vi "Store ASCII string.vi"(8 "error in (no error)":errorcluster, 10 "String to store (max 16 chars)":string, 11 "VISA resource name":refnum<visa-resource-name>) -> (0 "error out":errorcluster, 3 "VISA resource name out":refnum<visa-resource-name>)   [LabVIEW 2012, in "Datron D4xxx.lvlib"]
doc: "This VI stores 16 characters long string into instrument memory (I command)."
uses:
  Datron D4xxx.lvlib
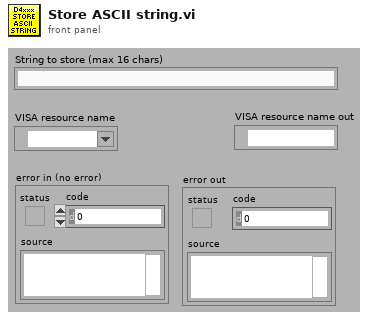
[diagram p1: front panel]
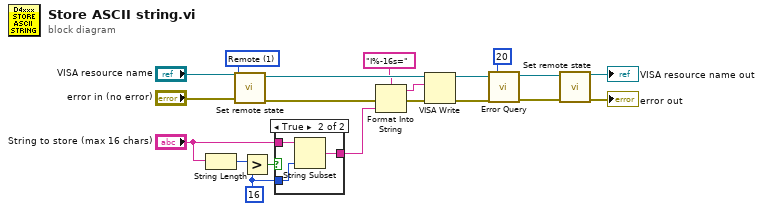
[diagram p0: block diagram]
diagram:
  w6 = 16 ("y")
  w16 = u16 1 items=["Local", "Remote", "Default"] ("Remote state")
  n1 = String Length(string="String to store (max 16 chars)") -> (length=w9:i32)
  n2 = call "Set remote state.vi"("error in"="error in (no error)", "Remote state"=w16, "VISA resource name"="VISA resource name") -> ("error out"=w14:errorcluster, "VISA resource name out"=w13:refnum<visa-resource-name>)  [unwired: 7 in]
  n3 = Greater?(x=w9, y=w6) -> (0:w10:bool)
  n4 = case shown="True" w10 {
    tunnel: "String to store (max 16 chars)" -> [w21 w24]
    tunnel: [w21 w23] -> w7
    tunnel: w6 -> [_ w22]
    frame False {
    }
    frame True {
      n5 = String Subset(string=w24, length (rest)=w22) -> (substring=w23:string)  [unwired: 1 in]
    }
  }
  n6 = Format Into String(format string="I%-16s=", error in=w14, w7) -> (resulting string=w11:string, error out=w15:errorcluster)  [unwired: 1 in]
  n7 = VISA Write(VISA resource name=w13, write buffer=w11, error in (no error)=w15) -> (VISA resource name out=w3:refnum<visa-resource-name>, error out=w5:errorcluster)  [unwired: 1 out]
  n8 = call "Error Query.vi"("error in (no error)"=w5, "Check cycles (11)"=20, "VISA resource name"=w3) -> ("error out"=w4:errorcluster, "VISA resource name out"=w2:refnum<visa-resource-name>)  [unwired: 5 in, 2 out]
  n9 = call "Set remote state.vi"("error in"=w4, "VISA resource name"=w2) -> ("error out"=→"error out":errorcluster, "VISA resource name out"=→"VISA resource name out":refnum<visa-resource-name>)  [unwired: 8 in]
